vi "ExecuteZeroing.vi"(8 "Error in":errorcluster, 9 "NumberOfMeasurementValuesToUse":i32=1, 11 "DevicesAndSignals":T1) -> (0 "Error out":errorcluster, 3 "DevicesAndSignals":T1)   [LabVIEW 2016]
doc: "Executes a zero balancing for all signals (notice that actually the channels zero offset will be set and therefore other signals that belong to the same channel are also affected).\n\nDevicesAndSignals: Array of devices and array of signals. Zeroing is done for all signals within the array. Zeroing can only be executed for signals that deliver valid measurement values!\nNumberOfMeasurementValuesToUse: Defines how many measurement values of each signal will be used to calculate an average mean value that will be used as zero offset for the signals (default value is 1)."
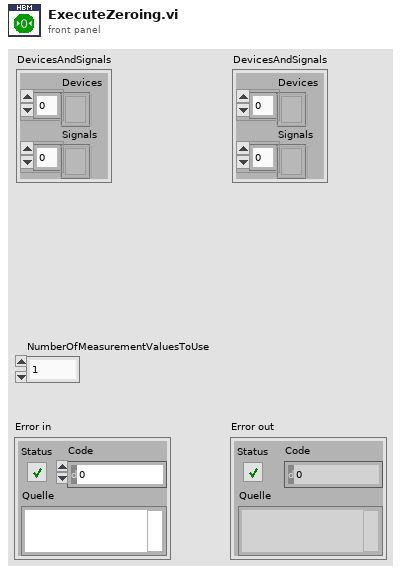
[diagram p1: front panel]
types:
  T1 = cluster{"Devices":refnum<k24>[], "Signals":refnum<k24>[]}
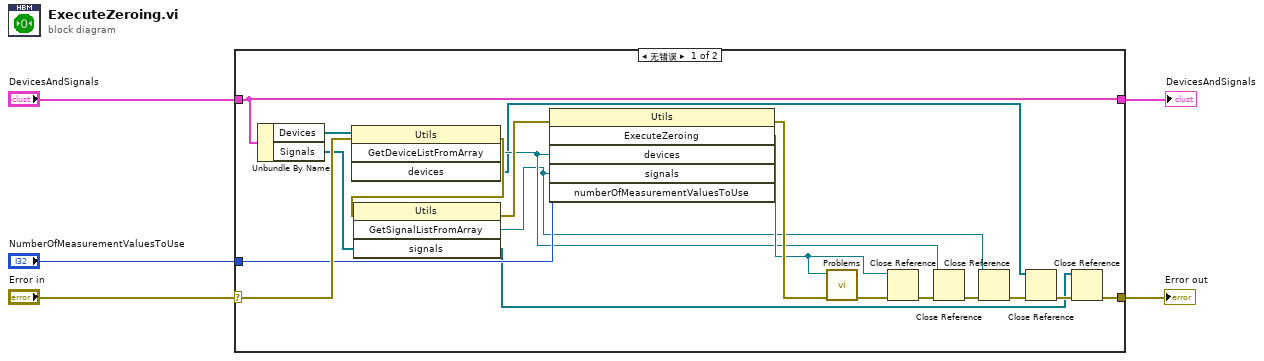
[diagram p0: block diagram]
diagram:
  n1 = case shown="无错误" "Error in" {
    selector: "Error in" -> [w23 w26]
    tunnel: "DevicesAndSignals" -> [w24 w25]
    tunnel: [w6 w26] -> w3
    tunnel: [w24 w25] -> w2
    tunnel: "NumberOfMeasurementValuesToUse" -> [w18 _]
    frame No Error {
      n2 = Unbundle By Name(w24) -> ("Devices"=w9:refnum<k24>[], "Signals"=w21:refnum<k24>[])
      n3 = invoke on="Methodenknoten" class="Utils" method="GetDeviceListFromArray"(error in=w23, "devices"=w9) -> (error out=w22:errorcluster, "GetDeviceListFromArray"=w14:refnum<k24>, "devices"=w8:refnum<k24>[])  [unwired: 2 in, 1 out]
      n4 = invoke on="Methodenknoten" class="Utils" method="GetSignalListFromArray"(error in=w22, "signals"=w21) -> (error out=w20:errorcluster, "GetSignalListFromArray"=w12:refnum<k24>, "signals"=w7:refnum<k24>[])  [unwired: 2 in, 1 out]
      n5 = invoke on="Methodenknoten" class="Utils" method="ExecuteZeroing"(error in=w20, "devices"=w14, "signals"=w12, "numberOfMeasurementValuesToUse"=w18) -> (error out=w19:errorcluster, "ExecuteZeroing"=w16:refnum<k24>)  [unwired: 2 in, 4 out]
      n6 = call "Problems.vi"("Error in"=w19, "Problems"=w16) -> ("Error out"=w17:errorcluster)  [unwired: 9 in]
      n7 = Close Reference(reference=w16, error in (no error)=w17) -> (error out=w15:errorcluster)
      n8 = Close Reference(reference=w14, error in (no error)=w15) -> (error out=w13:errorcluster)
      n9 = Close Reference(reference=w12, error in (no error)=w13) -> (error out=w11:errorcluster)
      n10 = Close Reference(reference=w8, error in (no error)=w11) -> (error out=w10:errorcluster)
      n11 = Close Reference(reference=w7, error in (no error)=w10) -> (error out=w6:errorcluster)
    }
    frame Error {
    }
  }
  "Error out" <- w3
  "DevicesAndSignals" <- w2
